vi "CSTK_MCListbox_Designer_InsertColHdr.vi"(7 "表头统一属性输入":refnum<vi>, 8 "错误输入（无错误）":errorcluster, 10 "MCListbox引用句柄":refnum<vi>, 11 "VI输入":refnum<vi>) -> (0 "错误输出":errorcluster, 3 "VI输出":refnum<vi>)   [LabVIEW 2015, in "CSTK_MCListbox Designer.lvlib"]
uses:
  CSTK_MCListbox Designer.lvlib
  _CSTK_MCListbox_Designer_ColHdr.ctl
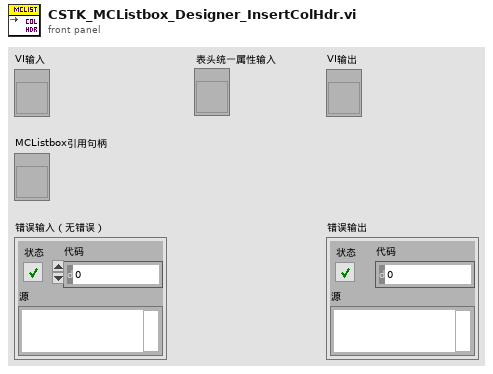
[diagram p1: front panel]
types:
  T1 = typedef "CSTK_MCListbox Designer.lvlib/_CSTK_MCListbox_Designer_ColHdr.ctl" = cluster{"列名称":string, "单元格宽度":u32, "粗体":bool, "斜体":bool, "对齐":enum16{"Left", "Center", "Right"}}
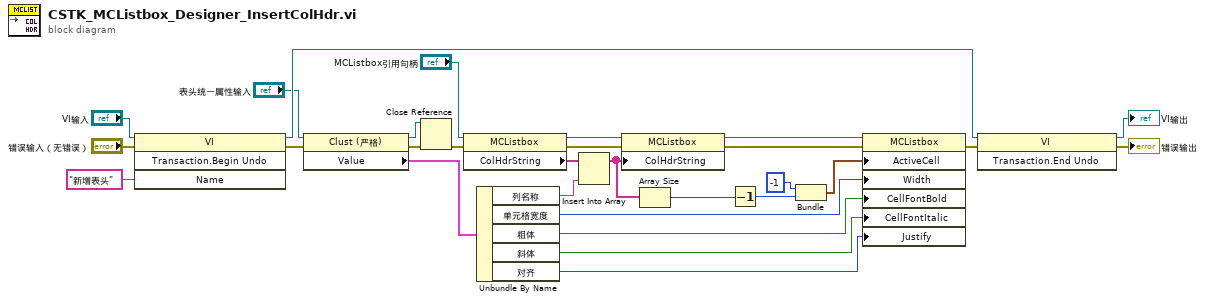
[diagram p0: block diagram]
diagram:
  n1 = invoke class="VI" method="Transaction.Begin Undo"(reference="VI输入", error in="错误输入（无错误）", "Name"="新增表头" ("名称")) -> (reference out=w9:refnum<vi>, error out=w8:errorcluster)  [unwired: 1 in, 2 out]
  n2 = property on="属性节点" class="Clust (严格)"(reference="表头统一属性输入", error in=w8) -> (reference out=w4:refnum<vi>, error out=w5:errorcluster, "Value"=w25:T1)
  n3 = Close Reference(reference=w4, error in (no error)=w5) -> (error out=w3:errorcluster)
  n4 = property class="MCListbox"(reference="MCListbox引用句柄", error in=w3) -> (reference out=w15:refnum<vi>, error out=w16:errorcluster, "ColHdrString"=w17:string[])
  n5 = Unbundle By Name(w25) -> ("列名称"=w7:string, "单元格宽度"=w24:u32, "粗体"=w26:bool, "斜体"=w1:bool, "对齐"=w27:enum16{"Left", "Center", "Right"})
  n6 = Insert Into Array(array=w17, new element=w7) -> (w21:string[])  [unwired: 1 in]
  n7 = property class="MCListbox"(reference=w15, error in=w16, "ColHdrString"=w21) -> (reference out=w18:refnum<vi>, error out=w6:errorcluster)
  n8 = Array Size(array=w21) -> (size(s)=w22:i32)
  n9 = Decrement(x=w22) -> (x-1=w23:i32)
  n10 = Bundle(-1, w23) -> (w20:cluster{i32, i32})  [unwired: 1 in]
  n11 = property class="MCListbox"(reference=w18, error in=w6, "ActiveCell"=w20, "Width"=w24, "CellFontBold"=w26, "CellFontItalic"=w1, "Justify"=w27) -> (error out=w28:errorcluster)  [unwired: 1 out]
  n12 = invoke class="VI" method="Transaction.End Undo"(reference=w9, error in=w28) -> (reference out=→"VI输出":refnum<vi>, error out=→"错误输出":errorcluster)  [unwired: 1 in, 1 out]
